vi "Access insert values.vi"(5 "是否创建唯一键":bool, 6 "Password":string, 7 "data":variant[](array[variant]), 8 "error in (no error)":errorcluster, 9 "columns外部输入":T1, 10 "database":string="database1.mdb", 11 "table":string) -> (0 "error out":errorcluster)   [LabVIEW 2022 SP3, in "Access Lib.lvlib"]
uses:
  Access Lib.lvlib
  <vilib>/addons/database/Auxilliary.llb/DB Tools Transaction.ctl
  <vilib>/addons/database/Auxilliary.llb/DB Tools Isolation Level.ctl
  <vilib>/addons/database/Auxilliary.llb/DB Tools Column Info.ctl
  <vilib>/addons/database/Auxilliary.llb/DB Tools DataTypes.ctl
  <vilib>/addons/database/Auxilliary.llb/DB Tools Parameter Info.ctl
  <vilib>/addons/database/Auxilliary.llb/DB Tools Parameter Dir.ctl
  <vilib>/addons/database/Connection.llb/DB Tools Open Connec (String).vi
  <vilib>/addons/database/Connection.llb/Conn Transaction.vi
  <vilib>/addons/database/Connection.llb/Conn Execute.vi
  <vilib>/addons/database/Recordset.llb/Rec Destroy - Connection.vi
  <vilib>/addons/database/Command.llb/Cmd Set Parameter Value (C).vi
  <vilib>/addons/database/Command.llb/Cmd Execute.vi
  <vilib>/addons/database/Recordset.llb/Rec Destroy - Command.vi
  <vilib>/addons/database/Command.llb/Cmd Delete.vi
  <vilib>/addons/database/NI_Database_API.lvlib
  <vilib>/Utility/VariantDataType/VariantType.lvlib
panel:
  out "当前数据时间":timestamp
  out "当前测量模式":string
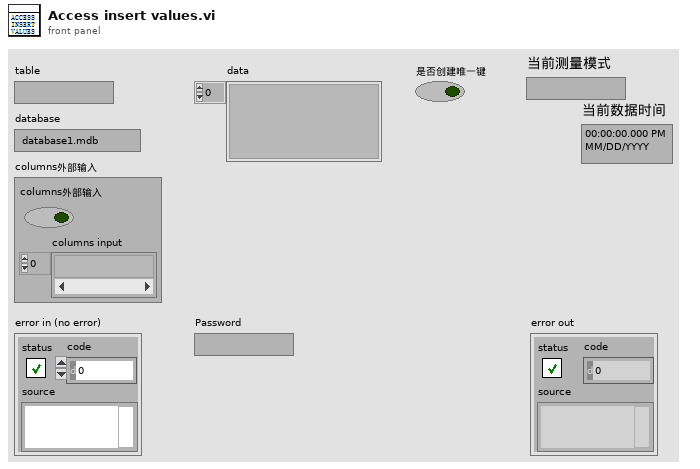
[diagram p1: front panel]
types:
  T1 = cluster{"columns外部输入":bool, "columns input":string[]}
  T2 = typedef "NI_Database_API.lvlib/DB Tools Isolation Level.ctl" = enum16{"chaos", "read uncommitted", "read committed", "repeatable read", "serializable"}
  T3 = typedef "NI_Database_API.lvlib/DB Tools Transaction.ctl" = enum16{"begin", "commit", "rollback"}
  T4 = typedef "NI_Database_API.lvlib/DB Tools Column Info.ctl" = cluster{"column name":string, "data type":T5, "size":i32, "allow null?":bool}
  T5 = typedef "NI_Database_API.lvlib/DB Tools DataTypes.ctl" = enum16{"String", "Long (I32)", "Single (SGL)", "Double (DBL)", "Date/Time", "Binary"}
  T6 = typedef "VariantType.lvlib/Type.ctl" = enum8{"Invalid Type", "Void", "I8", "I16", "I32", "I64", "U8", "U16", "U32", "U64", "Single Float", "Double Float", "Extended Float", "Single Complex", "Double Complex", "Extended Complex", "Enum U8", "Enum U16", "Enum U32", "Enum U64", "Single Float With Unit", "Double Float With Unit", "Extended Float With Unit", "Single Complex with Unit", "Double Complex with Unit", "Extended Complex with Unit", "Boolean", "String", "Path", "Picture", "Tag", "Array", "Cluster", "Variant", "LV Variant", "Waveform", "Timestamp", "Digital Waveform", "Digital Data", "ExpressData", "Refnum", "External Data", "VI", "Poly VI", "LabVIEW Class Instance", "Fixed Point"}
  T7 = typedef "NI_Database_API.lvlib/Conn ObjectReference.ctl" = refnum<k1>
  T8 = typedef "NI_Database_API.lvlib/DB Tools Parameter Info.ctl" = cluster{"parameter name":string, "type":T5, "direction":T9, "value":variant}
  T9 = typedef "NI_Database_API.lvlib/DB Tools Parameter Dir.ctl" = enum32{"Input", "Output", "Input/Output", "Return Value"}
  T10 = typedef "NI_Database_API.lvlib/Rec ObjectReference.ctl" = refnum<k1>
  T11 = typedef "LVDateTimeRec.ctl" = cluster{"秒数的小数部分":dbl, "秒":i32, "分":i32, "时":i32, "日":i32, "月":i32, "年":i32, "天数（周）":i32, "天数（年）":i32, "DST":i32}
  T12 = typedef "NI_Database_API.lvlib/Cmd ObjectReference.ctl" = refnum<k1>
  T13 = typedef "NI_Database_API.lvlib/Cmd-Rec Object Reference.ctl" = refnum<k1>
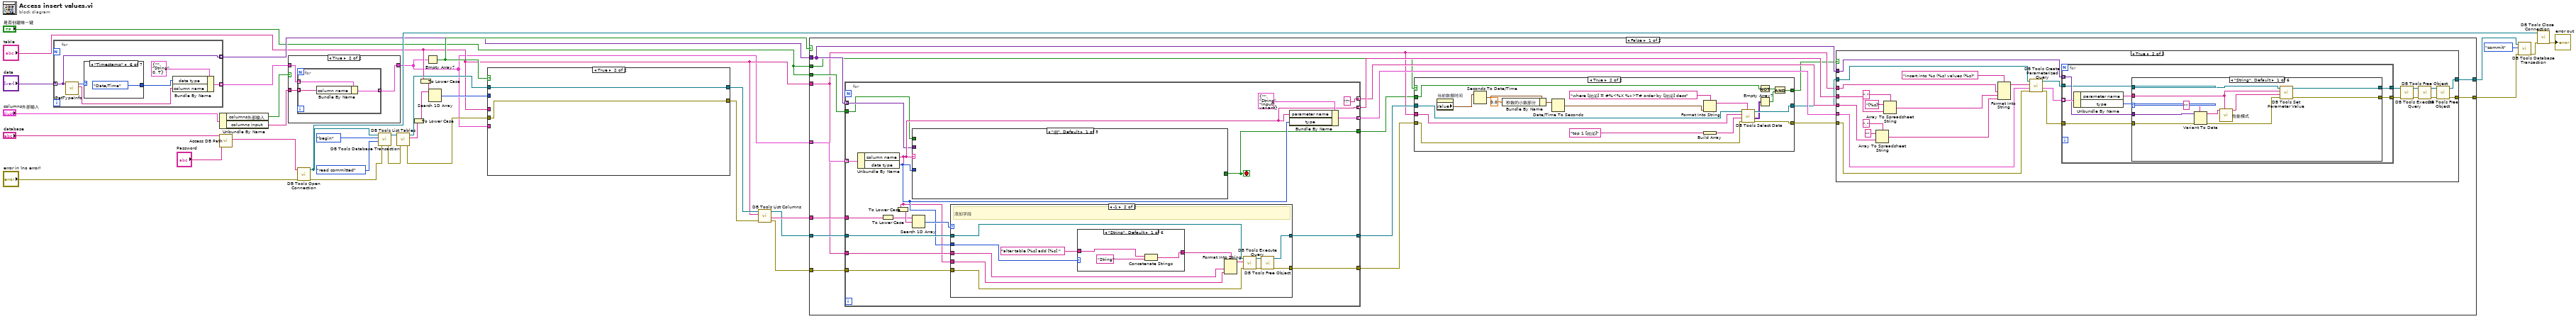
[diagram p0: block diagram]
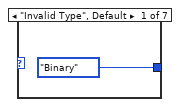
[diagram p3: hidden frame]
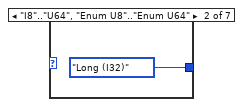
[diagram p4: hidden frame]
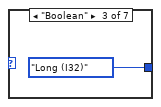
[diagram p5: hidden frame]
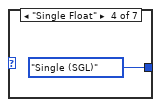
[diagram p6: hidden frame]
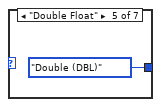
[diagram p7: hidden frame]
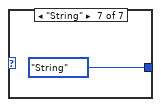
[diagram p8: hidden frame]
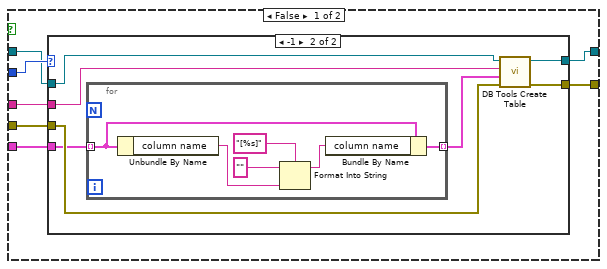
[diagram p9: hidden frame]
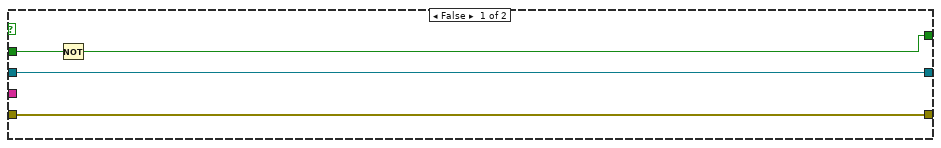
[diagram p11: hidden frame]
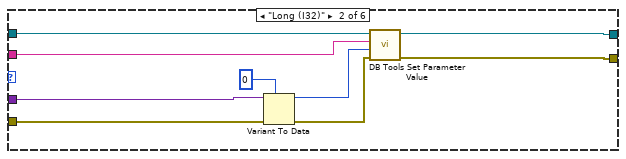
[diagram p13: hidden frame]
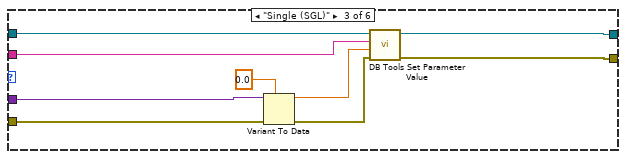
[diagram p14: hidden frame]
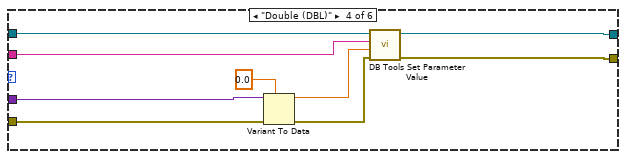
[diagram p15: hidden frame]
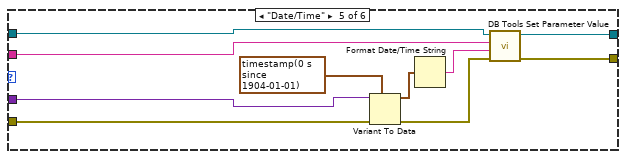
[diagram p16: hidden frame]
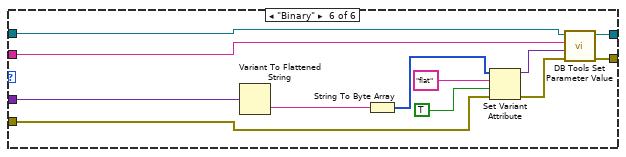
[diagram p17: hidden frame]
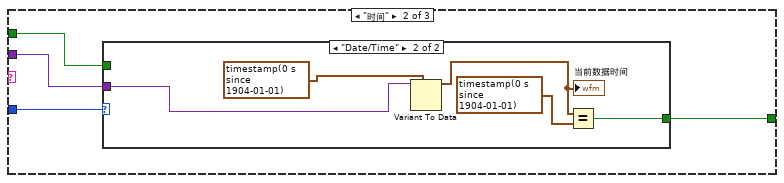
[diagram p18: hidden frame]
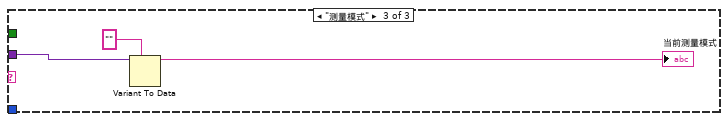
[diagram p20: hidden frame]
diagram:
  n1 = for {
    tunnel: [w37] -> w14 mode=indexing
    tunnel: [w39] -> w11 mode=indexing
    tunnel: "data" -> [w37] mode=indexing
    n2 = call <vilib>:"GetTypeInfo.vi"("Variant"=w37) -> ("Name"=w38:string, "Type Enum"=w41:T6)  [unwired: 6 in, 3 out]
    n3 = case shown="\"Timestamp\"" w41 {
      tunnel: [DB_Tools_DataTypes."Binary" ("data type") DB_Tools_DataTypes."Long (I32)" ("data type") DB_Tools_DataTypes."Long (I32)" ("data type") DB_Tools_DataTypes."Single (SGL)" ("data type") DB_Tools_DataTypes."Double (DBL)" ("data type") DB_Tools_DataTypes."Date/Time" ("data type") DB_Tools_DataTypes."String" ("data type")] -> w40
      frame "Invalid Type", Default {
      }
      frame "I8".."U64", "Enum U8".."Enum U64" {
      }
      frame "Boolean" {
      }
      frame "Single Float" {
      }
      frame "Double Float" {
      }
      frame "Timestamp" {
      }
      frame "String" {
      }
    }
    n4 = Bundle By Name(cluster=T4 {"column name"="", "data type"=enum."String", "size"=0, "allow null?"=TRUE} ("column information"), "data type"=w40, "column name"=w38) -> (w39:T4)
  }
  n5 = Unbundle By Name("columns外部输入") -> ("columns外部输入"=w9:bool, "columns input"=w10:string[])
  n6 = call "Access DB Path.vi"("Password"="Password", "database"="database") -> ("Connection information"=w7:string)  [unwired: 8 in, 1 out]
  n7 = case shown="True" w9 {
    tunnel: w11 -> [w50 w53]
    tunnel: [w50 w52] -> w8
    tunnel: w10 -> [_ w51]
    frame False {
    }
    frame True {
      n8 = for {
        tunnel: w53 -> [w56] mode=indexing
        tunnel: [w55] -> w52 mode=indexing
        tunnel: w51 -> [w54] mode=indexing
        n9 = Bundle By Name(cluster=w56, "column name"=w54) -> (w55:T4)
      }
    }
  }
  n10 = call-poly <vilib>:"DB Tools Open Connection.vi"("error in (no error)"="error in (no error)", "connection information"=w7) -> ("error out"=w21:errorcluster, "connection reference"=w18:T7)  [unwired: 6 in]
  n11 = call-poly <vilib>:"DB Tools Database Transaction.vi"("error in (no error)"=w21, "isolation level (chaos)"=DB_Tools_Isolation_Level."read committed", "operation (begin)"=DB_Tools_Transaction."begin", "connection reference"=w18) -> ("error out"=w20:errorcluster, "connection reference out"=w22:T7)  [unwired: 2 in]
  n12 = call <vilib>:"DB Tools List Tables.vi"("error in (no error)"=w20, "connection reference"=w22) -> ("error out"=w29:errorcluster, "tables"=w31:string[], "connection reference out"=w19:T7)  [unwired: 3 in]
  n13 = To Lower Case(string=w31) -> (all lower case string=w1:string[])
  n14 = To Lower Case(string="table") -> (all lower case string=w2:string)
  n15 = Empty Array?(array=w8) -> (empty?=w16:bool)
  n16 = Search 1D Array(1D array=w1, element=w2) -> (index of element=w30:i32)  [unwired: 1 in]
  n17 = case shown="True" w16 {
    tunnel: w30 -> [w63 _]
    tunnel: w29 -> [w62 w79]
    tunnel: [w61 w80] -> w27
    tunnel: [w60 w79] -> w26
    tunnel: w19 -> [w59 w80]
    tunnel: "table" -> [w58 _]
    tunnel: w8 -> [w57 _]
    frame False {
      n18 = case shown="-1" w63 {
        tunnel: w59 -> [w65 w72]
        tunnel: w62 -> [w64 w71]
        tunnel: w58 -> [_ w70]
        tunnel: w57 -> [_ w67]
        tunnel: [w65 w69] -> w61
        tunnel: [w64 w68] -> w60
        frame 0, Default {
        }
        frame -1 {
          n19 = for {
            tunnel: w67 -> [w74] mode=indexing
            tunnel: [w73] -> w66 mode=indexing
            n20 = Unbundle By Name(w74) -> ("column name"=w78:string)
            n21 = Format Into String(format string="[%s]" ("格式字符串"), initial string="" ("初始字符串"), w78) -> (resulting string=w75:string)  [unwired: 1 in, 1 out]
            n22 = Bundle By Name(cluster=w74, "column name"=w75) -> (w73:T4)
          }
          n23 = call <vilib>:"DB Tools Create Table.vi"("error in (no error)"=w71, "column information"=w66, "table"=w70, "connection reference"=w72) -> ("error out"=w68:errorcluster, "connection reference out"=w69:T7)  [unwired: 4 in]
        }
      }
    }
    frame True {
    }
  }
  n24 = call <vilib>:"DB Tools List Columns.vi"("error in (no error)"=w26, "table"="table", "connection reference"=w27) -> ("error out"=w5:errorcluster, "columns"=w28:string[], "connection reference out"=w6:T7)  [unwired: 1 in, 1 out]
  n25 = case shown="False" w16 {
    tunnel: w28 -> [w99 _]
    tunnel: w5 -> [w98 w280]
    tunnel: [w94 w281] -> w24
    tunnel: [w93 w280] -> w23
    tunnel: w14 -> [w90 _]
    tunnel: w6 -> [w92 w281]
    tunnel: "table" -> [w84 _]
    tunnel: w8 -> [w91 _]
    tunnel: "是否创建唯一键" -> [w89 _]
    tunnel: "是否创建唯一键" -> [w82 _]
    frame False {
      n26 = for {
        tunnel: w92 -> [w233]
        tunnel: w99 -> [w235]
        tunnel: w98 -> [w232]
        tunnel: [w231] -> w86
        tunnel: w84 -> [w230]
        tunnel: w91 -> [w229] mode=indexing
        tunnel: [w227] -> w97 mode=indexing
        tunnel: [w223] -> w96 mode=indexing
        tunnel: ["?"] -> w95 mode=indexing
        tunnel: [w225] -> w88
        tunnel: w90 -> [w222] mode=indexing
        tunnel: [w221] -> w83
        tunnel: w89 -> [w220]
        stop <- w221 stop-if-true
        n27 = Unbundle By Name(w229) -> ("column name"=w223:string, "data type"=w224:T5)
        n28 = To Lower Case(string=w235) -> (all lower case string=w218:string[])
        n29 = To Lower Case(string=w223) -> (all lower case string=w219:string)
        n30 = case shown="\"假\", Default" w223 {
          tunnel: w224 -> [_ w239 _]
          tunnel: w222 -> [_ w238 w247]
          tunnel: [_ w237 _] -> w221
          tunnel: w220 -> [_ w236 _]
          frame "假", Default {
          }
          frame "时间" {
            n31 = case shown="\"Date/Time\"" w239 {
              tunnel: w238 -> [_ w244]
              tunnel: [_ w240] -> w237
              tunnel: w236 -> [_ _]
              frame "String", Default {
              }
              frame "Date/Time" {
                n32 = Variant To Data(type=timestamp(0 s since 1904-01-01) ("时间标识"), Variant=w244) -> (data=w242:timestamp)  [unwired: 1 in, 1 out]
                "当前数据时间" <- w242
                n33 = Equal?(x=w242, y=timestamp(0 s since 1904-01-01) ("时间标识")) -> (x = y?=w240:bool)
              }
            }
          }
          frame "测量模式" {
            n34 = Variant To Data(type="", Variant=w247) -> (data=→"当前测量模式":string)  [unwired: 1 in, 1 out]
          }
        }
        n35 = Search 1D Array(1D array=w218, element=w219) -> (index of element=w234:i32)  [unwired: 1 in]
        n36 = case shown="-1" w234 {
          tunnel: [w249 w258] -> w231
          tunnel: w233 -> [w248 w257]
          tunnel: w223 -> [_ w256]
          tunnel: w232 -> [w249 w255]
          tunnel: w230 -> [_ w254]
          tunnel: w224 -> [_ w252]
          tunnel: [w248 w250] -> w225
          frame 0, Default {
          }
          frame -1 {
            # "添加字段"
            n37 = case shown="\"String\", Default" w252 {
              tunnel: "alter table [%s] add [%s] " -> [w264 w267 w270 w273 w276 w279]
              tunnel: [w263 w266 w269 w272 w275 w278] -> w251
              frame "String", Default {
                n38 = Concatenate Strings(w264, "String" ("字符串")) -> (w263:string)
              }
              frame "Long (I32)" {
                n39 = Concatenate Strings(w267, "Long" ("字符串")) -> (w266:string)
              }
              frame "Single (SGL)" {
                n40 = Concatenate Strings(w270, "Single" ("字符串")) -> (w269:string)
              }
              frame "Double (DBL)" {
                n41 = Concatenate Strings(w273, "Double" ("字符串")) -> (w272:string)
              }
              frame "Date/Time" {
                n42 = Concatenate Strings(w276, "TimeStamp" ("字符串")) -> (w275:string)
              }
              frame "Binary" {
                n43 = Concatenate Strings(w279, "Binary" ("字符串")) -> (w278:string)
              }
            }
            n44 = Format Into String(format string=w251, w254, w256) -> (resulting string=w259:string)  [unwired: 2 in, 1 out]
            n45 = call-poly <vilib>:"DB Tools Execute Query.vi"("error in (no error)"=w255, "SQL query"=w259, "connection reference"=w257) -> ("error out"=w260:errorcluster, "recordset reference"=w261:T10)  [unwired: 5 in]
            n46 = call-poly <vilib>:"DB Tools Free Object.vi"("error in (no error)"=w260, "recordset reference"=w261) -> ("error out"=w258:errorcluster, "connection reference"=w250:T7)  [unwired: 8 in]
          }
        }
        n47 = Bundle By Name(cluster=T8 {"parameter name"="", "type"=enum."String", "direction"=enum."Input", "value"=variant} ("parameter information"), "parameter name"=w223, "type"=w224) -> (w227:T8)
      }
      n48 = case shown="True" w82 {
        tunnel: w88 -> [w103 w120]
        tunnel: [w103 w119] -> w87
        tunnel: w86 -> [w102 w118]
        tunnel: [w102 w117] -> w85
        tunnel: w84 -> [_ w116]
        tunnel: w83 -> [w101 w105]
        tunnel: [w100 w107] -> w81
        frame False {
          n49 = Not(x=w101) -> (.not. x?=w100:bool)
        }
        frame True {
          n50 = property on="当前数据时间" class="AbsTime (strict)"() -> ("Value"=w113:timestamp)  [unwired: 2 in, 2 out]
          n51 = Seconds To Date/Time(time stamp (now)=w113) -> (date time rec=w112:T11)  [unwired: 1 in]
          n52 = Bundle By Name(cluster=w112, "秒数的小数部分"=0.0) -> (w109:T11)
          n53 = Date/Time To Seconds(2:w109) -> (0:w110:timestamp)  [unwired: 1 in]
          n54 = Format Into String(format string="where [时间] = #%<%X %x>T# order by [时间] desc" ("condition"), w110) -> (resulting string=w115:string)  [unwired: 2 in, 1 out]
          n55 = Build Array("top 1 [时间]") -> (w122:string[])
          n56 = call <vilib>:"DB Tools Select Data.vi"("condition"=w115, "error in (no error)"=w118, "columns"=w122, "table"=w116, "connection reference"=w120) -> ("error out"=w117:errorcluster, "data"=w108:variant[][], "connection reference out"=w119:T7)  [unwired: 1 in]
          n57 = Not(x=w105) -> (.not. x?=w104:bool)
          n58 = Empty Array?(array=w108) -> (empty?=w106:bool)
          n59 = And(x=w104, y=w106) -> (x .and. y?=w107:bool)
        }
      }
      n60 = case shown="True" w81 {
        tunnel: w97 -> [_ w150]
        tunnel: w96 -> [_ w144]
        tunnel: w95 -> [_ w142]
        tunnel: [w124 w132] -> w94
        tunnel: [w123 w131] -> w93
        tunnel: w87 -> [w124 w129]
        tunnel: w85 -> [w123 w127]
        tunnel: w84 -> [_ w126]
        tunnel: w90 -> [_ w125]
        frame False {
        }
        frame True {
          n61 = Array To Spreadsheet String(delimiter (Tab)="," ("分隔符(Tab)"), array=w142, 3:"" ("格式字符串")) -> (spreadsheet string=w141:string)
          n62 = Array To Spreadsheet String(delimiter (Tab)="," ("分隔符(Tab)"), array=w144, 3:"[%s]" ("格式字符串")) -> (spreadsheet string=w143:string)
          n63 = Format Into String(format string="insert into %s (%s) values (%s)" ("格式字符串"), w126, w143, w141) -> (resulting string=w140:string)  [unwired: 2 in, 1 out]
          n64 = call <vilib>:"DB Tools Create Parameterized Query.vi"("error in (no error)"=w127, "parameters"=w150, "SQL query"=w140, "connection reference"=w129) -> ("error out"=w139:errorcluster, "parameters out"=w138:T8[], "command reference"=w130:T12)  [unwired: 3 in]
          n65 = for {
            tunnel: w130 -> [w155]
            tunnel: w139 -> [w153]
            tunnel: w138 -> [w158] mode=indexing
            tunnel: w125 -> [w156] mode=indexing
            tunnel: [w152] -> w128
            tunnel: [w151] -> w137
            n66 = Unbundle By Name(w158) -> ("parameter name"=w154:string, "type"=w157:T5)
            n67 = case shown="\"String\", Default" w157 {
              tunnel: w156 -> [w165 w171 w178 w188 w205 w209]
              tunnel: w155 -> [w166 w175 w182 w192 w203 w217]
              tunnel: w154 -> [w159 w174 w181 w187 w198 w216]
              tunnel: w153 -> [w162 w169 w179 w189 w201 w208]
              tunnel: [w164 w173 w183 w191 w200 w215] -> w152
              tunnel: [w163 w172 w180 w190 w199 w214] -> w151
              frame "String", Default {
                n68 = Variant To Data(error in=w162, type="", Variant=w165) -> (data=w161:string, error out=w168:errorcluster)
                n69 = call "性能模式.vi"("colomn"=w159, "数据标识输入"=w161) -> ("数据标识输出"=w160:string)  [unwired: 9 in]
                n70 = call-poly <vilib>:"DB Tools Set Parameter Value.vi"("error in (no error)"=w168, "value"=w160, "parameter index"=w159, "command reference"=w166) -> ("error out"=w163:errorcluster, "command reference out"=w164:T12)  [unwired: 4 in]
              }
              frame "Long (I32)" {
                n71 = Variant To Data(error in=w169, type=0, Variant=w171) -> (data=w176:i32, error out=w177:errorcluster)
                n72 = call-poly <vilib>:"DB Tools Set Parameter Value.vi"("error in (no error)"=w177, "value"=w176, "parameter index"=w174, "command reference"=w175) -> ("error out"=w172:errorcluster, "command reference out"=w173:T12)  [unwired: 4 in]
              }
              frame "Single (SGL)" {
                n73 = Variant To Data(error in=w179, type=sgl 0.0, Variant=w178) -> (data=w185:sgl, error out=w186:errorcluster)
                n74 = call-poly <vilib>:"DB Tools Set Parameter Value.vi"("error in (no error)"=w186, "value"=w185, "parameter index"=w181, "command reference"=w182) -> ("error out"=w180:errorcluster, "command reference out"=w183:T12)  [unwired: 4 in]
              }
              frame "Double (DBL)" {
                n75 = Variant To Data(error in=w189, type=0.0, Variant=w188) -> (data=w194:dbl, error out=w195:errorcluster)
                n76 = call-poly <vilib>:"DB Tools Set Parameter Value.vi"("error in (no error)"=w195, "value"=w194, "parameter index"=w187, "command reference"=w192) -> ("error out"=w190:errorcluster, "command reference out"=w191:T12)  [unwired: 4 in]
              }
              frame "Date/Time" {
                n77 = Variant To Data(error in=w201, type=timestamp(0 s since 1904-01-01) ("时间标识"), Variant=w205) -> (data=w197:timestamp, error out=w202:errorcluster)
                n78 = Format Date/Time String(seconds (now)=w197) -> (date/time string=w196:string)  [unwired: 2 in]
                n79 = call-poly <vilib>:"DB Tools Set Parameter Value.vi"("error in (no error)"=w202, "value"=w196, "parameter index"=w198, "command reference"=w203) -> ("error out"=w199:errorcluster, "command reference out"=w200:T12)  [unwired: 4 in]
              }
              frame "Binary" {
                n80 = Variant To Flattened String(Variant=w209) -> (data string=w210:string)  [unwired: 1 out]
                n81 = String To Byte Array(string=w210) -> (unsigned byte array=w213:u8[])
                n82 = Set Variant Attribute(Variant=w213, name="flat", value=TRUE, error in=w208) -> (Variant out=w206:variant, error out=w207:errorcluster)  [unwired: 1 out]
                n83 = call-poly <vilib>:"DB Tools Set Parameter Value.vi"("error in (no error)"=w207, "value"=w206, "parameter index"=w216, "command reference"=w217) -> ("error out"=w214:errorcluster, "command reference out"=w215:T12)  [unwired: 4 in]
              }
            }
          }
          n84 = call-poly <vilib>:"DB Tools Execute Query.vi"("error in (no error)"=w137, "command reference"=w128) -> ("error out"=w135:errorcluster, "command-recordset reference"=w136:T13)  [unwired: 6 in]
          n85 = call-poly <vilib>:"DB Tools Free Object.vi"("error in (no error)"=w135, "command-recordset reference"=w136) -> ("error out"=w133:errorcluster, "command reference"=w134:T12)  [unwired: 8 in]
          n86 = call-poly <vilib>:"DB Tools Free Object.vi"("error in (no error)"=w133, "command reference"=w134) -> ("error out"=w131:errorcluster, "connection reference"=w132:T7)  [unwired: 8 in]
        }
      }
    }
    frame True {
    }
  }
  n87 = call-poly <vilib>:"DB Tools Database Transaction.vi"("error in (no error)"=w23, "operation (begin)"=DB_Tools_Transaction."commit", "connection reference"=w24) -> ("error out"=w25:errorcluster)  [unwired: 3 in, 1 out]
  n88 = call <vilib>:"DB Tools Close Connection.vi"("error in (no error)"=w25, "connection reference"=w18) -> ("error out"=→"error out":errorcluster)  [unwired: 5 in]
